vi "Simulation.vi"   [LabVIEW 2019]
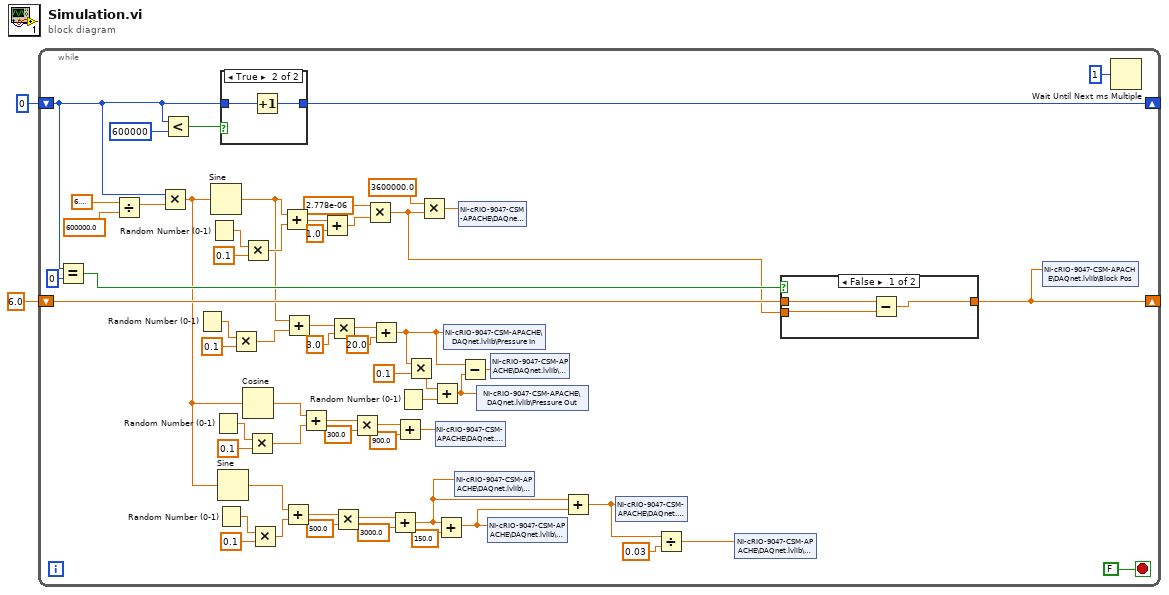
[diagram p0: block diagram]
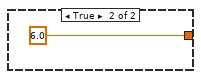
[diagram p2: hidden frame]
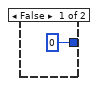
[diagram p3: hidden frame]
diagram:
  n1 = while {
    shift-right: [w60] -> _
    shift-left: 0 -> [w46]
    shift-right: [w43] -> _
    shift-left: 6.0 -> [w44]
    stop <- FALSE stop-if-true
    n2 = Equal?(x=w46, y=0) -> (x = y?=w47:bool)
    n3 = Divide(x=6.283185307179586, y=600000.0) -> (x/y=w57:dbl)
    n4 = Multiply(x=w46, y=w57) -> (x*y=w16:dbl)
    n5 = Less?(x=w46, y=600000) -> (x < y?=w61:bool)
    n6 = Random Number (0-1)() -> (number: 0 to 1=w41:dbl)
    n7 = Random Number (0-1)() -> (number: 0 to 1=w56:dbl)
    n8 = Sine(x=w16) -> (sin(x)=w39:dbl)
    n9 = Random Number (0-1)() -> (number: 0 to 1=w27:dbl)
    n10 = Random Number (0-1)() -> (number: 0 to 1=w18:dbl)
    n11 = Sine(x=w16) -> (sin(x)=w14:dbl)
    n12 = case shown="True" w61 {
      tunnel: w46 -> [_ w70]
      tunnel: [0 w69] -> w60
      frame False {
      }
      frame True {
        n13 = Increment(x=w70) -> (x+1=w69:i32)
      }
    }
    n14 = Multiply(x=w41, y=0.1) -> (x*y=w38:dbl)
    n15 = Multiply(x=w56, y=0.1) -> (x*y=w54:dbl)
    n16 = Cosine(x=w16) -> (cos(x)=w25:dbl)
    n17 = Multiply(x=w27, y=0.1) -> (x*y=w24:dbl)
    n18 = Multiply(x=w18, y=0.1) -> (x*y=w15:dbl)
    n19 = Add(x=w39, y=w54) -> (x+y=w53:dbl)
    n20 = Add(x=w14, y=w15) -> (x+y=w13:dbl)
    n21 = Add(x=w39, y=w38) -> (x+y=w37:dbl)
    n22 = Add(x=w25, y=w24) -> (x+y=w23:dbl)
    n23 = Add(x=w53, y=1.0) -> (x+y=w51:dbl)
    n24 = Multiply(x=w37, y=3.0) -> (x*y=w35:dbl)
    n25 = Multiply(x=w13, y=500.0) -> (x*y=w11:dbl)
    n26 = Multiply(x=w23, y=300.0) -> (x*y=w21:dbl)
    n27 = Multiply(x=2.778e-06, y=w51) -> (x*y=w42:dbl)
    n28 = Add(x=w35, y=20.0) -> (x+y=w30:dbl)
    n29 = Add(x=w11, y=3000.0) -> (x+y=w7:dbl)
    n30 = Add(x=w21, y=900.0) -> (x+y=w19:dbl)
    n31 = Random Number (0-1)() -> (number: 0 to 1=w31:dbl)
    n32 = Multiply(x=w30, y=0.1) -> (x*y=w32:dbl)
    n33 = Multiply(x=3600000.0, y=w42) -> (x*y=w49:dbl)
    n34 = Add(x=w32, y=w31) -> (x+y=w29:dbl)
    n35 = shared-variable "NI-cRIO-9047-CSM-APACHE\\DAQnet.lvlib\\RPM"(w19) -> ()  [unwired: 1 in, 1 out]
    n36 = Add(x=w7, y=150.0) -> (x+y=w8:dbl)
    n37 = shared-variable "NI-cRIO-9047-CSM-APACHE\\DAQnet.lvlib\\Pressure In"(w30) -> ()  [unwired: 1 in, 1 out]
    n38 = shared-variable "NI-cRIO-9047-CSM-APACHE\\DAQnet.lvlib\\Load 1"(w7) -> ()  [unwired: 1 in, 1 out]
    n39 = shared-variable "NI-cRIO-9047-CSM-APACHE\\DAQnet.lvlib\\ROP"(w49) -> ()  [unwired: 1 in, 1 out]
    n40 = Subtract(x=w30, y=w29) -> (x-y=w28:dbl)
    n41 = shared-variable "NI-cRIO-9047-CSM-APACHE\\DAQnet.lvlib\\Pressure Out"(w29) -> ()  [unwired: 1 in, 1 out]
    n42 = shared-variable "NI-cRIO-9047-CSM-APACHE\\DAQnet.lvlib\\Load 2"(w8) -> ()  [unwired: 1 in, 1 out]
    n43 = shared-variable "NI-cRIO-9047-CSM-APACHE\\DAQnet.lvlib\\DeltaP"(w28) -> ()  [unwired: 1 in, 1 out]
    n44 = Add(x=w7, y=w8) -> (x+y=w6:dbl)
    n45 = shared-variable "NI-cRIO-9047-CSM-APACHE\\DAQnet.lvlib\\WOB"(w6) -> ()  [unwired: 1 in, 1 out]
    n46 = Divide(x=w6, y=0.03 ("x/y")) -> (x/y=w4:dbl)
    n47 = shared-variable "NI-cRIO-9047-CSM-APACHE\\DAQnet.lvlib\\Torque"(w4) -> ()  [unwired: 1 in, 1 out]
    n48 = case shown="False" w47 {
      tunnel: w44 -> [w66 _]
      tunnel: [w64 6.0] -> w43
      tunnel: w42 -> [w65 _]
      frame False {
        n49 = Subtract(x=w66, y=w65) -> (x-y=w64:dbl)
      }
      frame True {
      }
    }
    n50 = shared-variable "NI-cRIO-9047-CSM-APACHE\\DAQnet.lvlib\\Block Pos"(w43) -> ()  [unwired: 1 in, 1 out]
    n51 = Wait Until Next ms Multiple(millisecond multiple=u32 1) -> ()  [unwired: 1 out]
  }
